vi "LoadParameters.vi"() -> (0 "Camera Control":T2={"Acquisition Freq"=30.0, "Exposure (ms)"=10.0, "Gain"=10.0, "Height"=1200, "Width"=2000, "Acq. trigger start"=TRUE} {"Acquisition Freq" min=1e-06 max=60.0; "Height" min=400 max=2064 step=1; "Width" min=400 max=3088 step=1}, 1 "Camera config":string)   [LabVIEW 2021]
panel:
  in  "Parameter name":T1={"Frame rate"="CameraAttributes::AcquisitionControl::AcquisitionFrameRate", "Gain"="CameraAttributes::AnalogControl::Gain", "Height"="CameraAttributes::ImageFormatControl::Height", "Width"="CameraAttributes::ImageFormatControl::Width", "Trigger"="CameraAttributes::AcquisitionControl::TriggerSelector = \"Frame Start\"\nCameraAttributes::AcquisitionControl::TriggerMode", "Exposure Time"="CameraAttributes::AcquisitionControl::ExposureTime"}
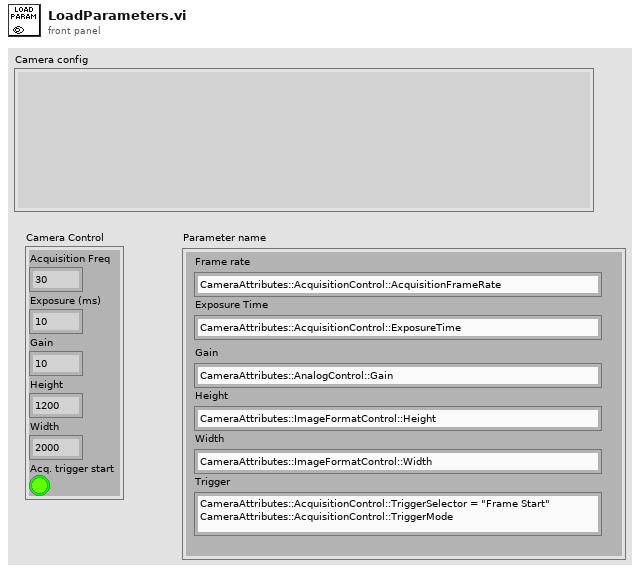
[diagram p1: front panel]
types:
  T1 = cluster{"Frame rate":string, "Gain":string, "Height":string, "Width":string, "Trigger":string, "Exposure Time":string}
  T2 = cluster{"Acquisition Freq":dbl, "Exposure (ms)":dbl, "Gain":sgl, "Height":u16, "Width":u16, "Acq. trigger start":bool}
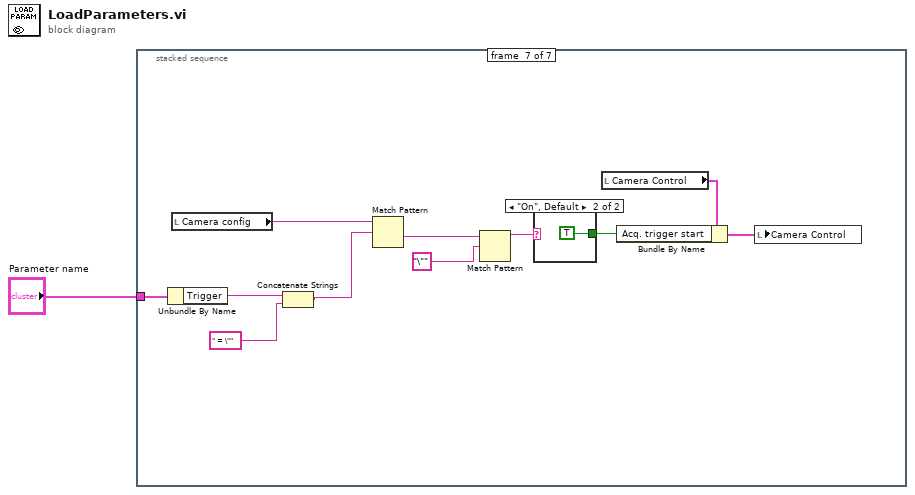
[diagram p0: block diagram]
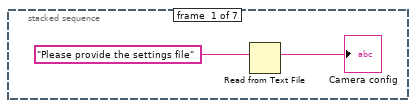
[diagram p2: hidden frame]
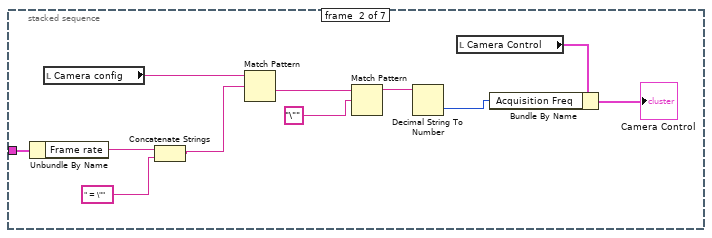
[diagram p3: hidden frame]
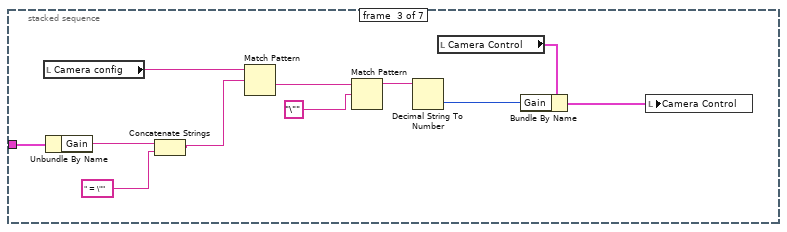
[diagram p4: hidden frame]
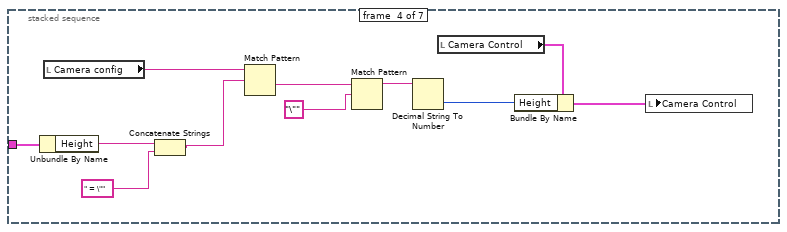
[diagram p5: hidden frame]
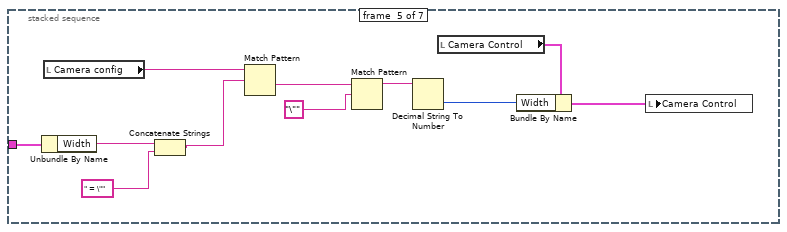
[diagram p6: hidden frame]
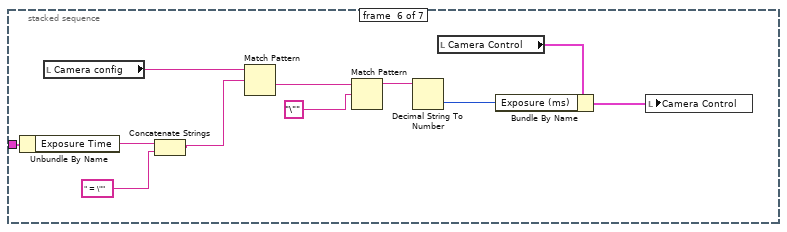
[diagram p7: hidden frame]
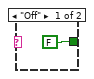
[diagram p8: hidden frame]
diagram:
  n1 = stacked-sequence {
    tunnel: "Parameter name" -> [_ w9 w20 w31 w42 w53 w64]
    frame #0 {
      n2 = Read from Text File(prompt (Open existing file)="Please provide the settings file") -> (text=→"Camera config":string)  [unwired: 3 in, 3 out]
    }
    frame #1 {
      n3 = Unbundle By Name(w9) -> ("Frame rate"=w8:string)
      n4 = local read "Camera config"() -> (w10:string)
      n5 = Concatenate Strings(w8, " = \"") -> (w13:string)
      n6 = Match Pattern(string=w10, regular expression=w13) -> (after substring=w14:string)  [unwired: 1 in, 3 out]
      n7 = Match Pattern(string=w14, regular expression="\"") -> (before substring=w7:string)  [unwired: 1 in, 3 out]
      n8 = Decimal String To Number(string=w7) -> (number=w4:i32)  [unwired: 2 in, 1 out]
      n9 = local read "Camera Control"() -> (w5:T2)
      n10 = Bundle By Name(cluster=w5, "Acquisition Freq"=w4) -> (→"Camera Control":T2)
    }
    frame #2 {
      n11 = local read "Camera config"() -> (w21:string)
      n12 = Unbundle By Name(w20) -> ("Gain"=w19:string)
      n13 = Concatenate Strings(w19, " = \"") -> (w24:string)
      n14 = Match Pattern(string=w21, regular expression=w24) -> (after substring=w25:string)  [unwired: 1 in, 3 out]
      n15 = Match Pattern(string=w25, regular expression="\"") -> (before substring=w18:string)  [unwired: 1 in, 3 out]
      n16 = Decimal String To Number(string=w18) -> (number=w16:i32)  [unwired: 2 in, 1 out]
      n17 = local read "Camera Control"() -> (w17:T2)
      n18 = Bundle By Name(cluster=w17, "Gain"=w16) -> (w15:T2)
      n19 = local write "Camera Control"(w15) -> ()
    }
    frame #3 {
      n20 = Unbundle By Name(w31) -> ("Height"=w30:string)
      n21 = local read "Camera config"() -> (w32:string)
      n22 = Concatenate Strings(w30, " = \"") -> (w35:string)
      n23 = Match Pattern(string=w32, regular expression=w35) -> (after substring=w36:string)  [unwired: 1 in, 3 out]
      n24 = Match Pattern(string=w36, regular expression="\"") -> (before substring=w29:string)  [unwired: 1 in, 3 out]
      n25 = Decimal String To Number(string=w29) -> (number=w27:i32)  [unwired: 2 in, 1 out]
      n26 = local read "Camera Control"() -> (w28:T2)
      n27 = Bundle By Name(cluster=w28, "Height"=w27) -> (w26:T2)
      n28 = local write "Camera Control"(w26) -> ()
    }
    frame #4 {
      n29 = Unbundle By Name(w42) -> ("Width"=w41:string)
      n30 = local read "Camera config"() -> (w43:string)
      n31 = Concatenate Strings(w41, " = \"") -> (w46:string)
      n32 = Match Pattern(string=w43, regular expression=w46) -> (after substring=w47:string)  [unwired: 1 in, 3 out]
      n33 = Match Pattern(string=w47, regular expression="\"") -> (before substring=w40:string)  [unwired: 1 in, 3 out]
      n34 = Decimal String To Number(string=w40) -> (number=w38:i32)  [unwired: 2 in, 1 out]
      n35 = local read "Camera Control"() -> (w39:T2)
      n36 = Bundle By Name(cluster=w39, "Width"=w38) -> (w37:T2)
      n37 = local write "Camera Control"(w37) -> ()
    }
    frame #5 {
      n38 = Unbundle By Name(w53) -> ("Exposure Time"=w52:string)
      n39 = local read "Camera config"() -> (w54:string)
      n40 = Concatenate Strings(w52, " = \"") -> (w57:string)
      n41 = Match Pattern(string=w54, regular expression=w57) -> (after substring=w58:string)  [unwired: 1 in, 3 out]
      n42 = Match Pattern(string=w58, regular expression="\"") -> (before substring=w51:string)  [unwired: 1 in, 3 out]
      n43 = Decimal String To Number(string=w51) -> (number=w49:i32)  [unwired: 2 in, 1 out]
      n44 = local read "Camera Control"() -> (w50:T2)
      n45 = Bundle By Name(cluster=w50, "Exposure (ms)"=w49) -> (w48:T2)
      n46 = local write "Camera Control"(w48) -> ()
    }
    frame #6 {
      n47 = Unbundle By Name(w64) -> ("Trigger"=w63:string)
      n48 = local read "Camera config"() -> (w65:string)
      n49 = Concatenate Strings(w63, " = \"") -> (w68:string)
      n50 = Match Pattern(string=w65, regular expression=w68) -> (after substring=w69:string)  [unwired: 1 in, 3 out]
      n51 = Match Pattern(string=w69, regular expression="\"") -> (before substring=w60:string)  [unwired: 1 in, 3 out]
      n52 = case shown="\"On\", Default" w60 {
        tunnel: [FALSE TRUE] -> w59
        frame "Off" {
        }
        frame "On", Default {
        }
      }
      n53 = local read "Camera Control"() -> (w62:T2)
      n54 = Bundle By Name(cluster=w62, "Acq. trigger start"=w59) -> (w61:T2)
      n55 = local write "Camera Control"(w61) -> ()
    }
  }
